vi "RTS Server Configuration.vi"(6 "Base Path":path, 7 "Index Number":i32=52, 8 "Error In":errorcluster, 11 "String Data":string[](array[string])) -> (0 "Error Out":errorcluster, 3 "Server Configuration":T1)   [LabVIEW 2016]
uses:
  Type Definitions/RTS Server Configuration.ctl
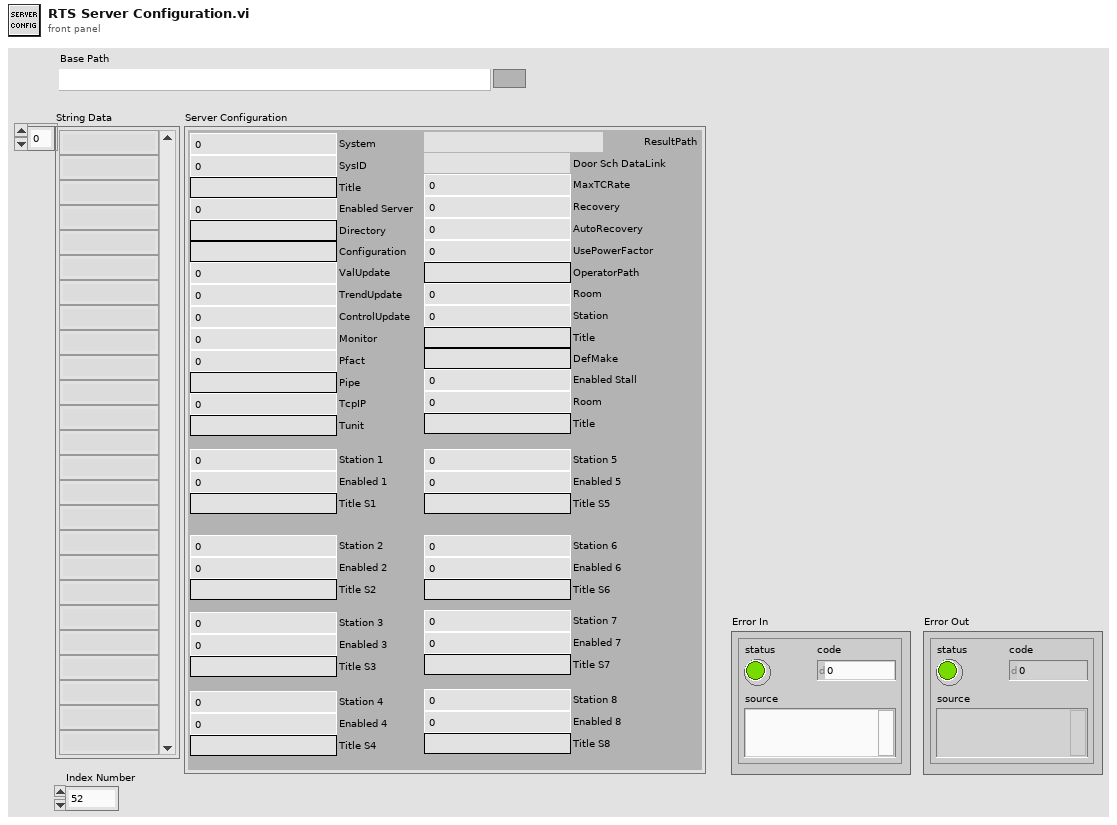
[diagram p1: front panel]
types:
  T1 = typedef "RTS Server Configuration.ctl" = cluster{"System":u16, "SysID":u16, "Title":string, "Enabled Server":u16, "Directory":string, "Configuration":string, "ValUpdate":u16, "TrendUpdate":u16, "ControlUpdate":u16, "Monitor":u16, "Pfact":u16, "Pipe":string, "TcpIP":u16, "Tunit":string, "ResultPath":path, "Door Sch DataLink":path, "MaxTCRate":u16, "Recovery":u16, "AutoRecovery":u16, "UsePowerFactor":u16, "OperatorPath":string, "Room":u16, "Station":u16, "Title":string, "DefMake":string, "Enabled Stall":u16, "Room":u16, "Title":string, "Station 1":u16, "Enabled 1":u16, "Station 2":u16, "Enabled 2":u16, "Station 3":u16, "Enabled 3":u16, "Station 4":u16, "Enabled 4":u16, "Station 5":u16, "Enabled 5":u16, "Station 6":u16, "Enabled 6":u16, "Station 7":u16, "Enabled 7":u16, "Station 8":u16, "Enabled 8":u16, "Title S1":string, "Title S2":string, "Title S3":string, "Title S5":string, "Title S6":string, "Title S7":string, "Title S8":string, "Title S4":string}
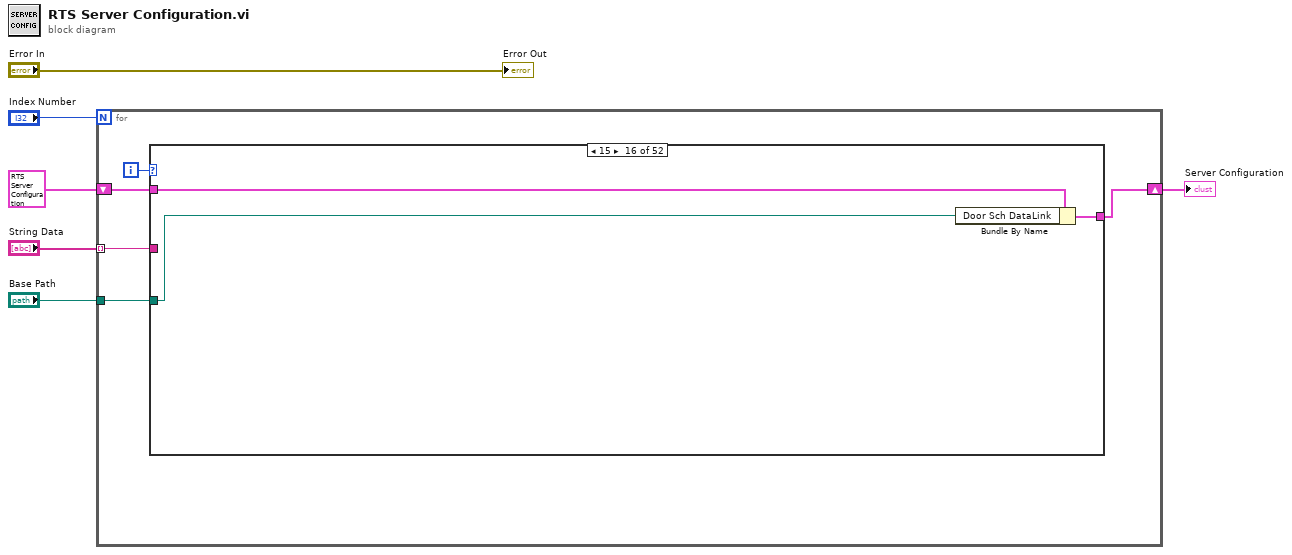
[diagram p0: block diagram]
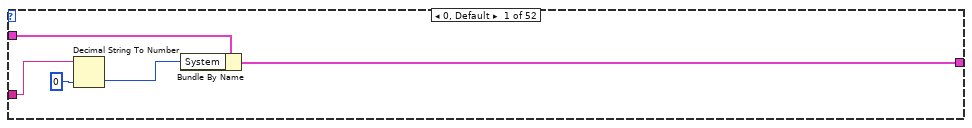
[diagram p2: hidden frame]
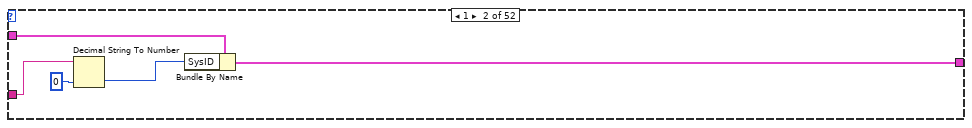
[diagram p3: hidden frame]
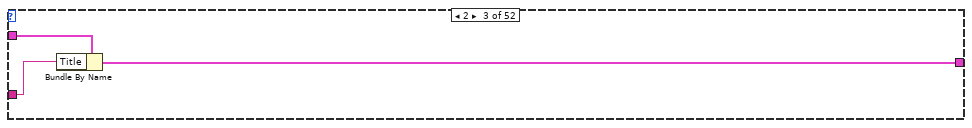
[diagram p4: hidden frame]
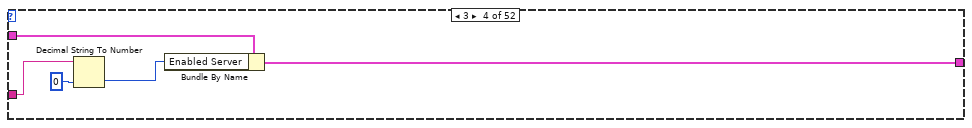
[diagram p5: hidden frame]
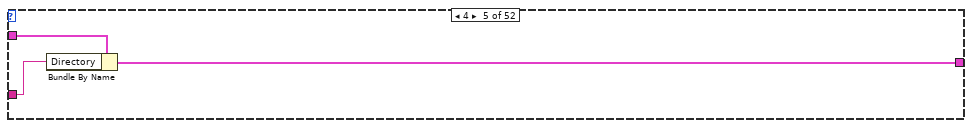
[diagram p6: hidden frame]
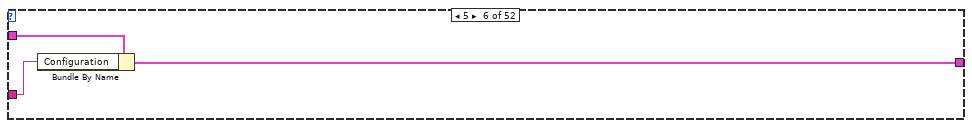
[diagram p7: hidden frame]
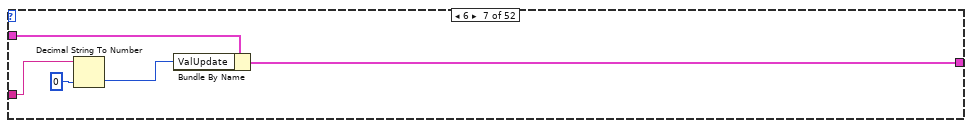
[diagram p8: hidden frame]
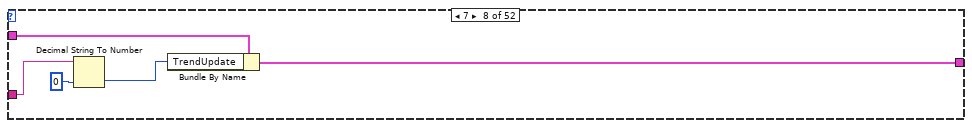
[diagram p9: hidden frame]
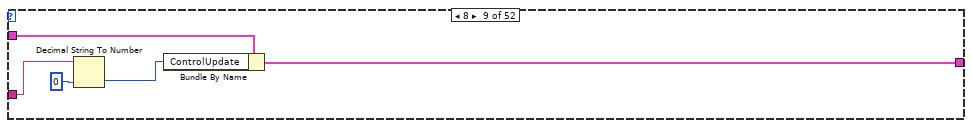
[diagram p10: hidden frame]
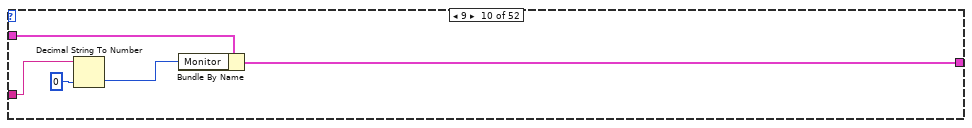
[diagram p11: hidden frame]
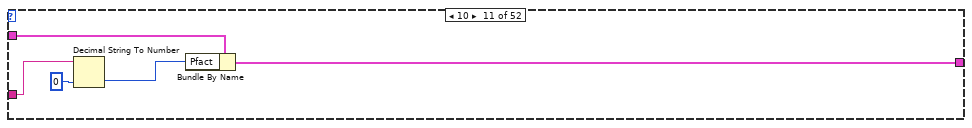
[diagram p12: hidden frame]
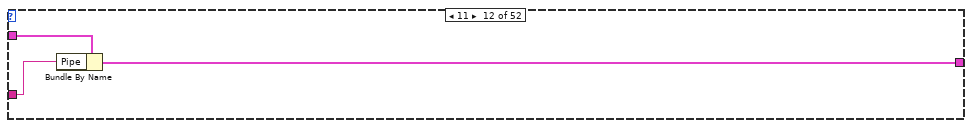
[diagram p13: hidden frame]
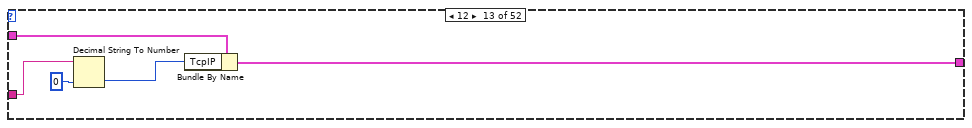
[diagram p14: hidden frame]
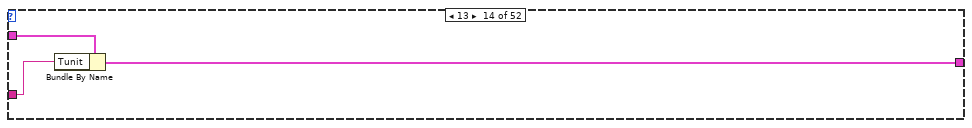
[diagram p15: hidden frame]
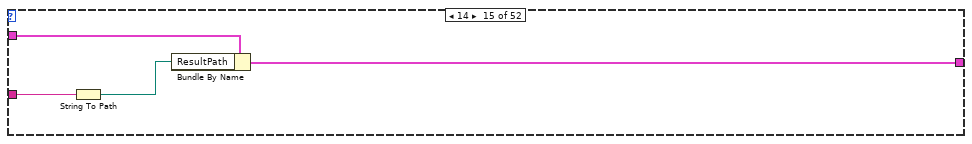
[diagram p16: hidden frame]
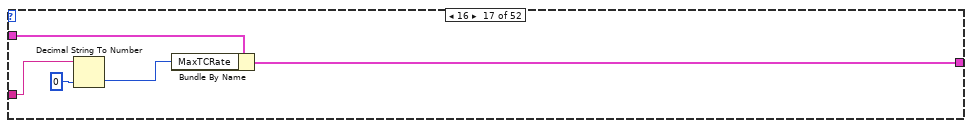
[diagram p17: hidden frame]
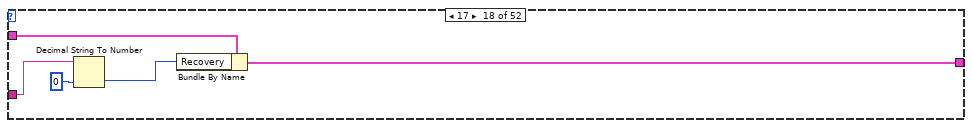
[diagram p18: hidden frame]
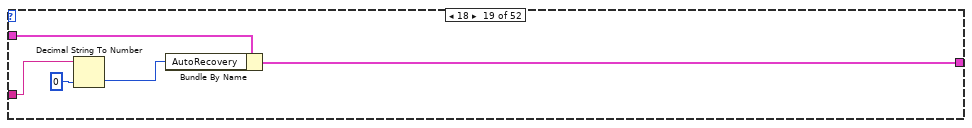
[diagram p19: hidden frame]
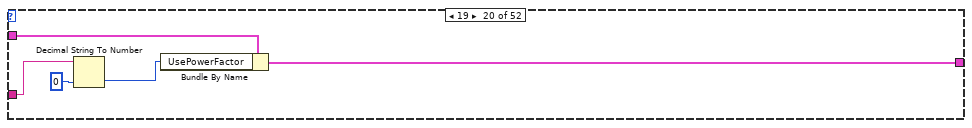
[diagram p20: hidden frame]
diagram:
  n1 = for {
    N: "Index Number" -> [_]
    tunnel: "String Data" -> [w10] mode=indexing
    shift-right: [w8] -> w6
    shift-left: T1 {"System"=0, "SysID"=0, "Title"="", "Enabled Server"=0, "Directory"="", "Configuration"="", "ValUpdate"=0, "TrendUpdate"=0, "ControlUpdate"=0, "Monitor"=0, "Pfact"=0, "Pipe"="", "TcpIP"=0, "Tunit"="", "ResultPath"=path "", "Door Sch DataLink"=path "", "MaxTCRate"=0, "Recovery"=0, "AutoRecovery"=0, "UsePowerFactor"=0, "OperatorPath"="", "Room"=0, "Station"=0, "Title"="", "DefMake"="", "Enabled Stall"=0, "Room"=0, "Title"="", "Station 1"=0, "Enabled 1"=0, "Station 2"=0, "Enabled 2"=0, "Station 3"=0, "Enabled 3"=0, "Station 4"=0, "Enabled 4"=0, "Station 5"=0, "Enabled 5"=0, "Station 6"=0, "Enabled 6"=0, "Station 7"=0, "Enabled 7"=0, "Station 8"=0, "Enabled 8"=0, "Title S1"="", "Title S2"="", "Title S3"="", "Title S5"="", "Title S6"="", "Title S7"="", "Title S8"="", "Title S4"=""} ("Server Configuration") -> [w9]
    tunnel: "Base Path" -> [w7]
    i -> [w11]
    n2 = case shown="15" w11 {
      tunnel: w10 -> [w14 w17 w22 w25 w30 w33 w36 w41 w46 w51 w56 w61 w65 w69 w74 _ w80 w85 w90 w95 w99 w103 w108 w112 w115 w119 w124 w128 w131 w136 w140 w144 w149 w152 w157 w162 w166 w171 w175 w178 w183 w188 w191 w196 w201 w204 w209 w214 w217 w222 w227 w230]
      tunnel: w9 -> [w16 w19 w24 w27 w32 w35 w38 w43 w48 w53 w58 w63 w68 w71 w75 w78 w83 w88 w93 w98 w101 w106 w111 w114 w117 w122 w127 w130 w135 w138 w143 w148 w151 w156 w161 w164 w169 w174 w177 w181 w185 w190 w193 w198 w203 w206 w211 w216 w219 w224 w229 w232]
      tunnel: [w15 w18 w23 w26 w31 w34 w37 w42 w47 w52 w57 w62 w67 w70 w72 w77 w82 w87 w92 w97 w100 w105 w110 w113 w116 w121 w126 w129 w134 w137 w142 w147 w150 w155 w160 w163 w168 w173 w176 w180 w184 w189 w192 w197 w202 w205 w210 w215 w218 w223 w228 w231] -> w8
      tunnel: w7 -> [_ _ _ _ _ _ _ _ _ _ _ _ _ _ _ w76 _ _ _ _ _ _ _ _ _ _ _ _ _ _ _ _ _ _ _ _ _ _ _ _ _ _ _ _ _ _ _ _ _ _ _ _]
      frame 0, Default {
        n3 = Decimal String To Number(string=w14, default (0L)=u16 0 ("default (0 I32)")) -> (number=w13:u16)  [unwired: 1 in, 1 out]
        n4 = Bundle By Name(cluster=w16, "System"=w13) -> (w15:T1)
      }
      frame 1 {
        n5 = Decimal String To Number(string=w17, default (0L)=u16 0 ("default (0 I32)")) -> (number=w21:u16)  [unwired: 1 in, 1 out]
        n6 = Bundle By Name(cluster=w19, "SysID"=w21) -> (w18:T1)
      }
      frame 2 {
        n7 = Bundle By Name(cluster=w24, "Title"=w22) -> (w23:T1)
      }
      frame 3 {
        n8 = Decimal String To Number(string=w25, default (0L)=u16 0 ("default (0 I32)")) -> (number=w29:u16)  [unwired: 1 in, 1 out]
        n9 = Bundle By Name(cluster=w27, "Enabled Server"=w29) -> (w26:T1)
      }
      frame 4 {
        n10 = Bundle By Name(cluster=w32, "Directory"=w30) -> (w31:T1)
      }
      frame 5 {
        n11 = Bundle By Name(cluster=w35, "Configuration"=w33) -> (w34:T1)
      }
      frame 6 {
        n12 = Decimal String To Number(string=w36, default (0L)=u16 0 ("default (0 I32)")) -> (number=w40:u16)  [unwired: 1 in, 1 out]
        n13 = Bundle By Name(cluster=w38, "ValUpdate"=w40) -> (w37:T1)
      }
      frame 7 {
        n14 = Decimal String To Number(string=w41, default (0L)=u16 0 ("default (0 I32)")) -> (number=w45:u16)  [unwired: 1 in, 1 out]
        n15 = Bundle By Name(cluster=w43, "TrendUpdate"=w45) -> (w42:T1)
      }
      frame 8 {
        n16 = Decimal String To Number(string=w46, default (0L)=u16 0 ("default (0 I32)")) -> (number=w50:u16)  [unwired: 1 in, 1 out]
        n17 = Bundle By Name(cluster=w48, "ControlUpdate"=w50) -> (w47:T1)
      }
      frame 9 {
        n18 = Decimal String To Number(string=w51, default (0L)=u16 0 ("default (0 I32)")) -> (number=w55:u16)  [unwired: 1 in, 1 out]
        n19 = Bundle By Name(cluster=w53, "Monitor"=w55) -> (w52:T1)
      }
      frame 10 {
        n20 = Decimal String To Number(string=w56, default (0L)=u16 0 ("default (0 I32)")) -> (number=w60:u16)  [unwired: 1 in, 1 out]
        n21 = Bundle By Name(cluster=w58, "Pfact"=w60) -> (w57:T1)
      }
      frame 11 {
        n22 = Bundle By Name(cluster=w63, "Pipe"=w61) -> (w62:T1)
      }
      frame 12 {
        n23 = Decimal String To Number(string=w65, default (0L)=u16 0 ("default (0 I32)")) -> (number=w64:u16)  [unwired: 1 in, 1 out]
        n24 = Bundle By Name(cluster=w68, "TcpIP"=w64) -> (w67:T1)
      }
      frame 13 {
        n25 = Bundle By Name(cluster=w71, "Tunit"=w69) -> (w70:T1)
      }
      frame 14 {
        n26 = String To Path(string=w74) -> (path=w73:path)
        n27 = Bundle By Name(cluster=w75, "ResultPath"=w73) -> (w72:T1)
      }
      frame 15 {
        n28 = Bundle By Name(cluster=w78, "Door Sch DataLink"=w76) -> (w77:T1)
      }
      frame 16 {
        n29 = Decimal String To Number(string=w80, default (0L)=u16 0 ("default (0 I32)")) -> (number=w79:u16)  [unwired: 1 in, 1 out]
        n30 = Bundle By Name(cluster=w83, "MaxTCRate"=w79) -> (w82:T1)
      }
      frame 17 {
        n31 = Decimal String To Number(string=w85, default (0L)=u16 0 ("default (0 I32)")) -> (number=w84:u16)  [unwired: 1 in, 1 out]
        n32 = Bundle By Name(cluster=w88, "Recovery"=w84) -> (w87:T1)
      }
      frame 18 {
        n33 = Decimal String To Number(string=w90, default (0L)=u16 0 ("default (0 I32)")) -> (number=w89:u16)  [unwired: 1 in, 1 out]
        n34 = Bundle By Name(cluster=w93, "AutoRecovery"=w89) -> (w92:T1)
      }
      frame 19 {
        n35 = Decimal String To Number(string=w95, default (0L)=u16 0 ("default (0 I32)")) -> (number=w94:u16)  [unwired: 1 in, 1 out]
        n36 = Bundle By Name(cluster=w98, "UsePowerFactor"=w94) -> (w97:T1)
      }
      frame 20 {
        n37 = Bundle By Name(cluster=w101, "OperatorPath"=w99) -> (w100:T1)
      }
      frame 21 {
        n38 = Decimal String To Number(string=w103, default (0L)=u16 0 ("default (0 I32)")) -> (number=w102:u16)  [unwired: 1 in, 1 out]
        n39 = Bundle By Name(cluster=w106, "Room"=w102) -> (w105:T1)
      }
      frame 22 {
        n40 = Decimal String To Number(string=w108, default (0L)=u16 0 ("default (0 I32)")) -> (number=w107:u16)  [unwired: 1 in, 1 out]
        n41 = Bundle By Name(cluster=w111, "Station"=w107) -> (w110:T1)
      }
      frame 23 {
        n42 = Bundle By Name(cluster=w114, "Title"=w112) -> (w113:T1)
      }
      frame 24 {
        n43 = Bundle By Name(cluster=w117, "DefMake"=w115) -> (w116:T1)
      }
      frame 25 {
        n44 = Decimal String To Number(string=w119, default (0L)=u16 0 ("default (0 I32)")) -> (number=w118:u16)  [unwired: 1 in, 1 out]
        n45 = Bundle By Name(cluster=w122, "Enabled Stall"=w118) -> (w121:T1)
      }
      frame 26 {
        n46 = Decimal String To Number(string=w124, default (0L)=u16 0 ("default (0 I32)")) -> (number=w123:u16)  [unwired: 1 in, 1 out]
        n47 = Bundle By Name(cluster=w127, "Room"=w123) -> (w126:T1)
      }
      frame 27 {
        n48 = Bundle By Name(cluster=w130, "Title"=w128) -> (w129:T1)
      }
      frame 28 {
        n49 = Decimal String To Number(string=w131, default (0L)=u16 0 ("default (0 I32)")) -> (number=w132:u16)  [unwired: 1 in, 1 out]
        n50 = Bundle By Name(cluster=w135, "Station 1"=w132) -> (w134:T1)
      }
      frame 29 {
        n51 = Bundle By Name(cluster=w138, "Title S1"=w136) -> (w137:T1)
      }
      frame 30 {
        n52 = Decimal String To Number(string=w140, default (0L)=u16 0 ("default (0 I32)")) -> (number=w139:u16)  [unwired: 1 in, 1 out]
        n53 = Bundle By Name(cluster=w143, "Enabled 1"=w139) -> (w142:T1)
      }
      frame 31 {
        n54 = Decimal String To Number(string=w144, default (0L)=u16 0 ("default (0 I32)")) -> (number=w145:u16)  [unwired: 1 in, 1 out]
        n55 = Bundle By Name(cluster=w148, "Station 2"=w145) -> (w147:T1)
      }
      frame 32 {
        n56 = Bundle By Name(cluster=w151, "Title S2"=w149) -> (w150:T1)
      }
      frame 33 {
        n57 = Decimal String To Number(string=w152, default (0L)=u16 0 ("default (0 I32)")) -> (number=w153:u16)  [unwired: 1 in, 1 out]
        n58 = Bundle By Name(cluster=w156, "Enabled 2"=w153) -> (w155:T1)
      }
      frame 34 {
        n59 = Decimal String To Number(string=w157, default (0L)=u16 0 ("default (0 I32)")) -> (number=w158:u16)  [unwired: 1 in, 1 out]
        n60 = Bundle By Name(cluster=w161, "Station 3"=w158) -> (w160:T1)
      }
      frame 35 {
        n61 = Bundle By Name(cluster=w164, "Title S3"=w162) -> (w163:T1)
      }
      frame 36 {
        n62 = Decimal String To Number(string=w166, default (0L)=u16 0 ("default (0 I32)")) -> (number=w165:u16)  [unwired: 1 in, 1 out]
        n63 = Bundle By Name(cluster=w169, "Enabled 3"=w165) -> (w168:T1)
      }
      frame 37 {
        n64 = Decimal String To Number(string=w171, default (0L)=u16 0 ("default (0 I32)")) -> (number=w170:u16)  [unwired: 1 in, 1 out]
        n65 = Bundle By Name(cluster=w174, "Station 4"=w170) -> (w173:T1)
      }
      frame 38 {
        n66 = Bundle By Name(cluster=w177, "Title S4"=w175) -> (w176:T1)
      }
      frame 39 {
        n67 = Decimal String To Number(string=w178, default (0L)=u16 0 ("default (0 I32)")) -> (number=w179:u16)  [unwired: 1 in, 1 out]
        n68 = Bundle By Name(cluster=w181, "Enabled 4"=w179) -> (w180:T1)
      }
      frame 40 {
        n69 = Decimal String To Number(string=w183, default (0L)=u16 0 ("default (0 I32)")) -> (number=w186:u16)  [unwired: 1 in, 1 out]
        n70 = Bundle By Name(cluster=w185, "Station 5"=w186) -> (w184:T1)
      }
      frame 41 {
        n71 = Bundle By Name(cluster=w190, "Title S5"=w188) -> (w189:T1)
      }
      frame 42 {
        n72 = Decimal String To Number(string=w191, default (0L)=u16 0 ("default (0 I32)")) -> (number=w194:u16)  [unwired: 1 in, 1 out]
        n73 = Bundle By Name(cluster=w193, "Enabled 5"=w194) -> (w192:T1)
      }
      frame 43 {
        n74 = Decimal String To Number(string=w196, default (0L)=u16 0 ("default (0 I32)")) -> (number=w199:u16)  [unwired: 1 in, 1 out]
        n75 = Bundle By Name(cluster=w198, "Station 6"=w199) -> (w197:T1)
      }
      frame 44 {
        n76 = Bundle By Name(cluster=w203, "Title S6"=w201) -> (w202:T1)
      }
      frame 45 {
        n77 = Decimal String To Number(string=w204, default (0L)=u16 0 ("default (0 I32)")) -> (number=w207:u16)  [unwired: 1 in, 1 out]
        n78 = Bundle By Name(cluster=w206, "Enabled 6"=w207) -> (w205:T1)
      }
      frame 46 {
        n79 = Decimal String To Number(string=w209, default (0L)=u16 0 ("default (0 I32)")) -> (number=w212:u16)  [unwired: 1 in, 1 out]
        n80 = Bundle By Name(cluster=w211, "Station 7"=w212) -> (w210:T1)
      }
      frame 47 {
        n81 = Bundle By Name(cluster=w216, "Title S7"=w214) -> (w215:T1)
      }
      frame 48 {
        n82 = Decimal String To Number(string=w217, default (0L)=u16 0 ("default (0 I32)")) -> (number=w220:u16)  [unwired: 1 in, 1 out]
        n83 = Bundle By Name(cluster=w219, "Enabled 7"=w220) -> (w218:T1)
      }
      frame 49 {
        n84 = Decimal String To Number(string=w222, default (0L)=u16 0 ("default (0 I32)")) -> (number=w225:u16)  [unwired: 1 in, 1 out]
        n85 = Bundle By Name(cluster=w224, "Station 8"=w225) -> (w223:T1)
      }
      frame 50 {
        n86 = Bundle By Name(cluster=w229, "Title S8"=w227) -> (w228:T1)
      }
      frame 51 {
        n87 = Decimal String To Number(string=w230, default (0L)=u16 0 ("default (0 I32)")) -> (number=w233:u16)  [unwired: 1 in, 1 out]
        n88 = Bundle By Name(cluster=w232, "Enabled 8"=w233) -> (w231:T1)
      }
    }
  }
  "Server Configuration" <- w6
  "Error Out" <- "Error In"
